vi "datasets.list.vi"(8 "error in":errorcluster, 11 "asset in":refnum<class "asset.lvclass">) -> (0 "error out":errorcluster, 2 "datasets":map{string, refnum<class "dataset.lvclass">}(c390), 3 "asset out":refnum<class "asset.lvclass">)   [LabVIEW 2020, in "asset.lvclass"]
doc: "Returns all datasets from an asset."
uses:
  asset.lvclass
  datasources/dataset/dataset.lvclass
  asset.lvclass/asset.ctl
  datascopes.get.vi
  Nominal Client/Nominal Client.lvclass
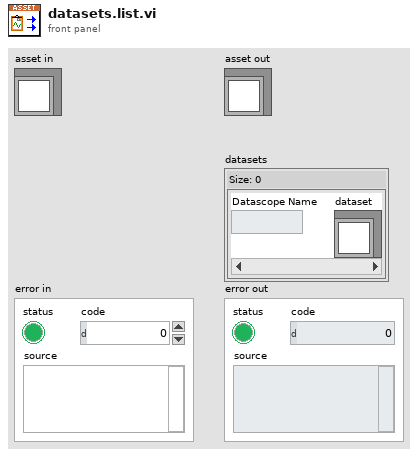
[diagram p1: front panel]
types:
  T1 = typedef "dataScopes.lvlib/data_scopes.ctl" = T2[]
  T2 = typedef "dataScopes.lvlib/data_scope.ctl" = cluster{"dataScopeName":string, "dataSource":T3, "seriesTags":map{string, string}, "offset":T5}
  T3 = typedef "dataScopes.lvlib/data_source.ctl" = cluster{"type":T4, "rid":string}
  T4 = typedef "dataScopes.lvlib/type.ctl" = enum16{"dataset", "connection", "logSet", "video"}
  T5 = typedef "dataScopes.lvlib/offset.ctl" = cluster{"seconds":i32, "nanos":i32, "picos":i32}
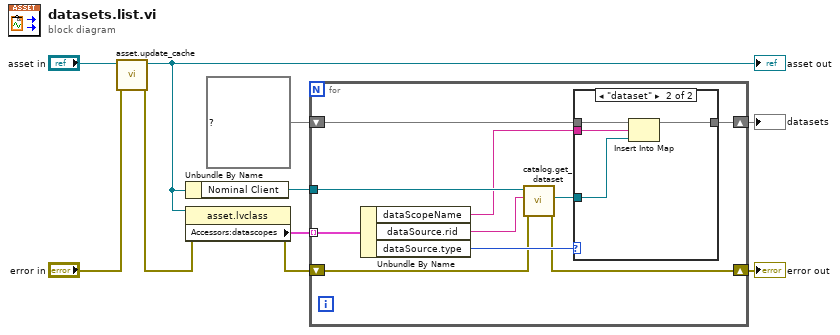
[diagram p0: block diagram]
diagram:
  n1 = call "asset.update_cache.vi"("error in"="error in", "asset in"="asset in") -> ("error out"=w7:errorcluster, "asset out"=w2:refnum<class "asset.lvclass">)  [unwired: 8 in]
  "asset out" <- w2
  n2 = Unbundle By Name(w2) -> ("Nominal Client"=w1:refnum<class "Nominal Client.lvclass">)
  n3 = property class="asset.lvclass"(reference=w2, error in=w7) -> (error out=w4:errorcluster, "Accessors:datascopes"=w10:T1)  [unwired: 1 out]
  n4 = for {
    tunnel: w10 -> [w20] mode=indexing
    shift-right: [w17] -> w5
    shift-left: map{string, refnum<class "dataset.lvclass">} {} ("map in") -> [w18]
    shift-right: [w14] -> w3
    shift-left: w4 -> [w15]
    tunnel: w1 -> [w12]
    n5 = Unbundle By Name(w20) -> ("dataScopeName"=w11:string, "dataSource.rid"=w16:string, "dataSource.type"=w19:T4)
    n6 = call "catalog.get_dataset.vi"("error in"=w15, "Dataset RID"=w16, "Nominal Client in"=w12) -> ("error out"=w14:errorcluster, "Dataset"=w13:refnum<class "dataset.lvclass">)  [unwired: 6 in, 1 out]
    n7 = case shown="\"dataset\"" w19 {
      tunnel: w18 -> [w21 w25]
      tunnel: [w21 w24] -> w17
      tunnel: w11 -> [_ w23]
      tunnel: w13 -> [_ w22]
      frame Default {
      }
      frame "dataset" {
        n8 = Insert Into Map(map in=w25, key=w23, value=w22) -> (map out=w24:map{string, refnum<class "dataset.lvclass">})  [unwired: 2 out]
      }
    }
  }
  "error out" <- w3
  "datasets" <- w5
